vi "testInsertOutOfRangeHigh.vi"(8 "error in (no error)":errorcluster, 11 "TestCase in":refnum<class "ListImp_Common.lvclass">) -> (0 "error out":errorcluster, 3 "TestCase out":refnum<class "ListImp_Common.lvclass">)   [LabVIEW 2013, in "ListImp_Common.lvclass"]
uses:
  ListImp_Common.lvclass
  ListImp_Common.lvclass/ListImp_Common.ctl
  source/LapDog.Collections.Lists/ListImp/ListImp.lvclass
  <vilib>/addons/_JKI Toolkits/VI Tester/TestCase.llb/TestCase.lvclass
  UnitTestComparisons/UnitTestComparisons.lvlib
  source/LapDog.Collections.Common/I32/I32.lvclass
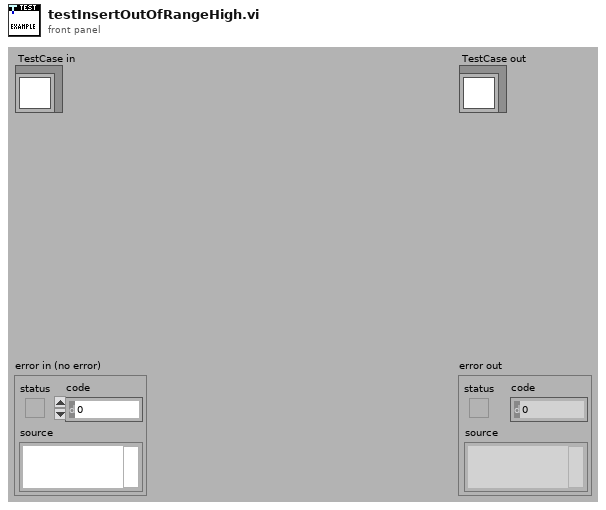
[diagram p1: front panel]
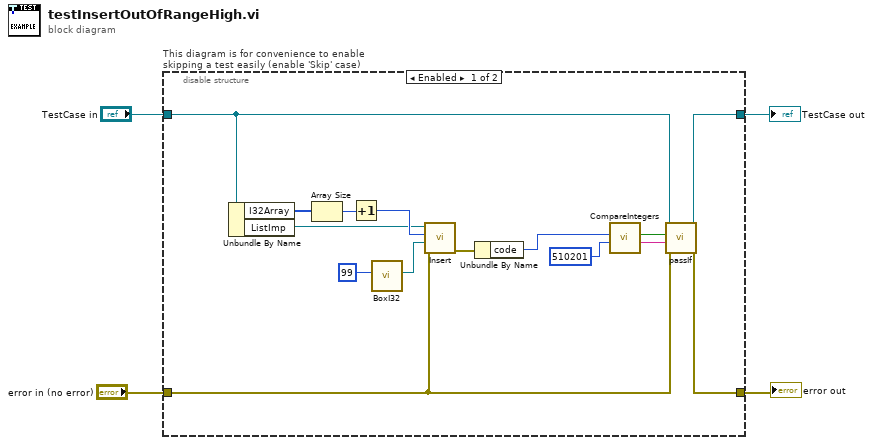
[diagram p0: block diagram]
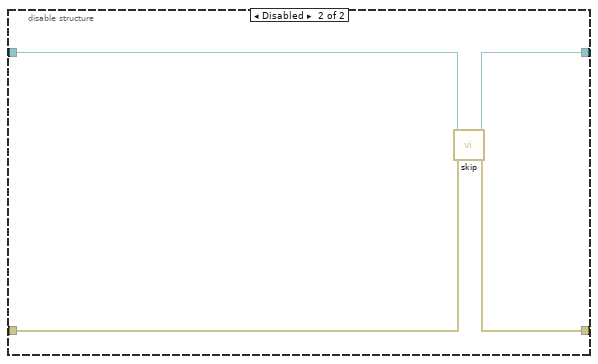
[diagram p2: hidden frame]
diagram:
  n1 = disable-structure "This diagram is for convenience to enable skipping a test easily (enable 'Skip' case)" shown="Enabled" {
    disable-tunnel: "TestCase in" -> [w17 w23]
    disable-tunnel: [w19 w21] -> w1
    disable-tunnel: [w18 w22] -> w3
    disable-tunnel: "error in (no error)" -> [w5 w20]
    frame Enabled {
      n2 = Unbundle By Name(w17) -> ("I32Array"=w7:i32[], "ListImp"=w8:refnum<class "ListImp.lvclass">)
      n3 = Array Size(array=w7) -> (size(s)=w6:i32)
      n4 = Increment(x=w6) -> (x+1=w9:i32)
      n5 = call "BoxI32.vi"("Numeric"=99) -> ("I32 out"=w10:refnum<class "I32.lvclass">)  [unwired: 10 in]
      n6 = call-dynamic "Insert.vi"("error in (no error)"=w5, "Item"=w10, "Index"=w9, "ListImp in"=w8) -> ("error out"=w13:errorcluster)  [unwired: 6 in, 1 out]
      n7 = Unbundle By Name(w13) -> ("code"=w12:i32)
      n8 = call "CompareIntegers.vi"("Expected Value"=510201, "Actual Value"=w12) -> ("Message"=w15:string, "Equal?"=w16:bool)  [unwired: 8 in]
      n9 = call-dynamic "passIf.vi"("error in (no error)"=w5, "message (\"\")"=w15, "pass"=w16, "TestCase in"=w17) -> ("error out"=w18:errorcluster, "TestCase out"=w19:refnum<class "ListImp_Common.lvclass">)  [unwired: 6 in]
    }
    frame Disabled {
      # "skip test result while test is under development"
      n10 = call <vilib>:"skip.vi"("error in (no error)"=w20, "TestCase in"=w23) -> ("error out"=w22:errorcluster, "TestCase out"=w21:refnum<class "ListImp_Common.lvclass">)  [unwired: 8 in]
    }
  }
  "error out" <- w3
  "TestCase out" <- w1
